vi "Get Terminal Refs for Response SubVI.vi"(8 "error in (no error)":errorcluster, 10 "object refnum":refnum<vi>, 11 "Getter Generator In":refnum<class "Getter Generator.lvclass">) -> (0 "error out":errorcluster, 2 "reference out":refnum<vi>, 3 "Getter Generator Out":refnum<class "Getter Generator.lvclass">)   [LabVIEW 2020, in "Method Generation.lvlib" / "Getter Generator.lvclass"]
uses:
  Getter Generator.lvclass
  Getter Generator.lvclass/Getter Generator.ctl
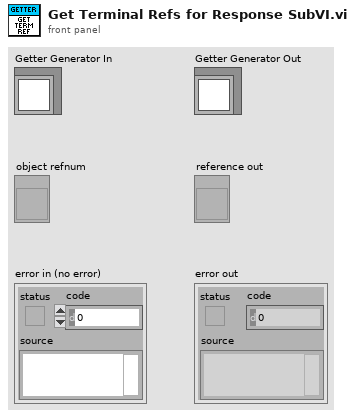
[diagram p1: front panel]
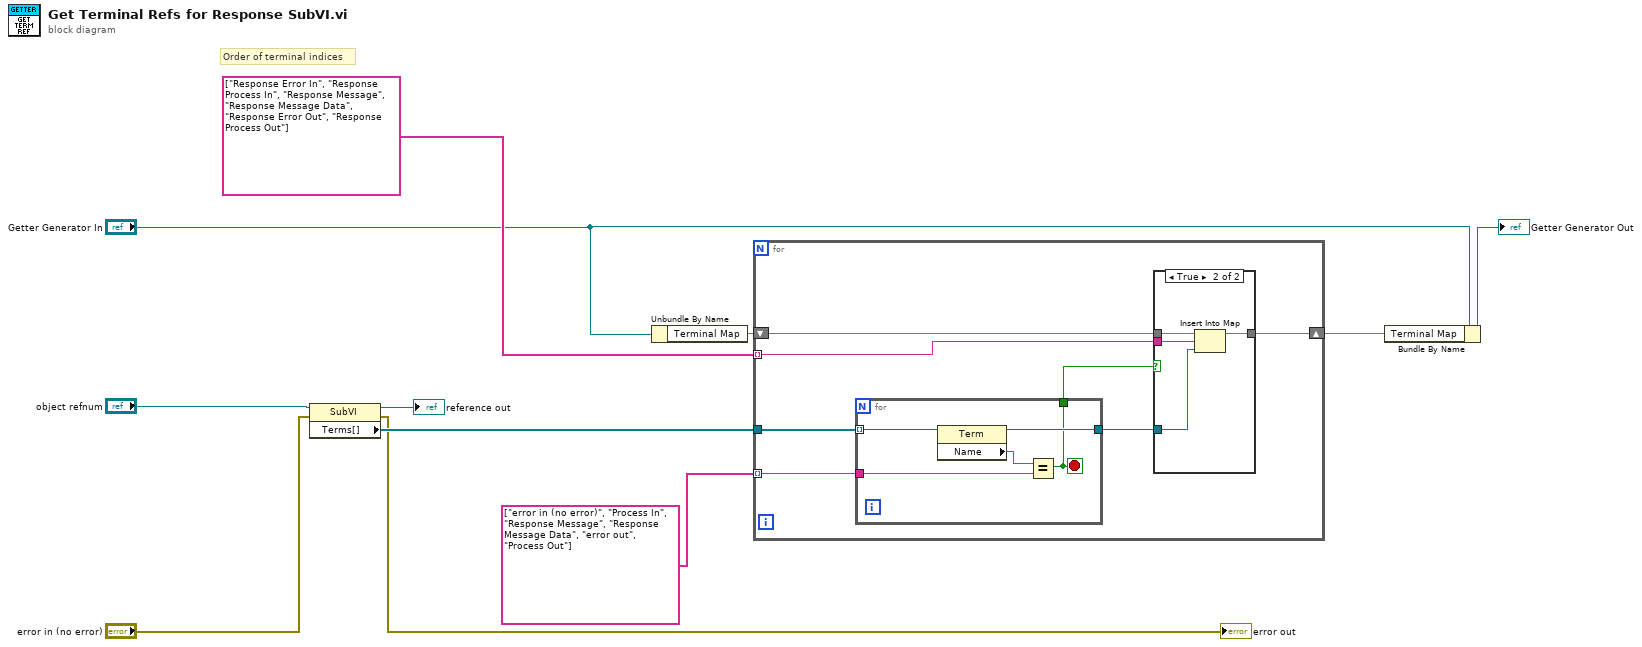
[diagram p0: block diagram]
diagram:
  # "Order of terminal indices"
  n1 = property class="SubVI"(reference="object refnum", error in="error in (no error)") -> (reference out=→"reference out":refnum<vi>, error out=→"error out":errorcluster, "Terms[]"=w10:refnum<vi>[])
  n2 = Unbundle By Name("Getter Generator In") -> ("Terminal Map"=w6:map{string, refnum<vi>})
  n3 = for {
    tunnel: w10 -> [w15]
    tunnel: string[] ["Response Error In", "Response Process In", "Response Message", "Response Message Data", "Response Error Out", "Response Process Out"] -> [w17] mode=indexing
    shift-right: [w16] -> w5
    shift-left: w6 -> [w18]
    tunnel: string[] ["error in (no error)", "Process In", "Response Message", "Response Message Data", "error out", "Process Out"] -> [w14] mode=indexing
    n4 = for {
      tunnel: w15 -> [w28] mode=indexing
      tunnel: [w27] -> w13
      tunnel: w14 -> [w25]
      tunnel: [w24] -> w12
      stop <- w24 stop-if-true
      n5 = property class="Term"(reference=w28) -> (reference out=w27:refnum<vi>, "Name"=w26:string)  [unwired: 1 in, 1 out]
      n6 = Equal?(x=w26, y=w25) -> (x = y?=w24:bool)
    }
    n7 = case shown="True" w12 {
      tunnel: w18 -> [w19 w23]
      tunnel: w17 -> [_ w22]
      tunnel: [w19 w21] -> w16
      tunnel: w13 -> [_ w20]
      frame False {
      }
      frame True {
        n8 = Insert Into Map(map in=w23, key=w22, value=w20) -> (map out=w21:map{string, refnum<vi>})  [unwired: 2 out]
      }
    }
  }
  n9 = Bundle By Name(cluster="Getter Generator In", "Terminal Map"=w5) -> (→"Getter Generator Out":refnum<class "Getter Generator.lvclass">)
